vi "LVClass_ClosedLoopSecurity_Dtor.vi"(0 "ClosedLoopSecurity in":refnum<class "ClosedLoopSecurity.lvclass">, 11 "error in (no error)":errorcluster) -> (4 "ClosedLoopSecurity out":refnum<class "ClosedLoopSecurity.lvclass">, 15 "error out":errorcluster)   [LabVIEW 2020, in "ClosedLoopSecurity.lvclass"]
doc: "Destruction.\n\n<B>security_paramsIn</B> : Pointer to threaded loop object.\n<B>security_paramsOut</B> : Pointer to threaded loop object."
uses:
  ClosedLoopSecurity.lvclass
  ClosedLoopSecurity.lvclass/ClosedLoopSecurity.ctl
  Controls/Handle creation.ctl
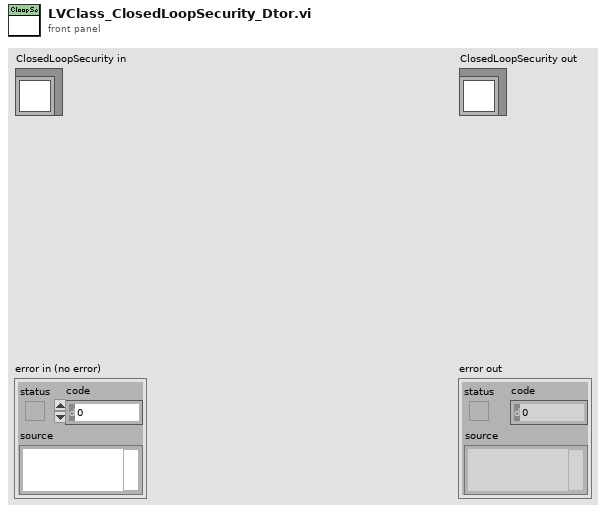
[diagram p1: front panel]
types:
  T1 = typedef "Handle creation.ctl" = enum16{"By ctor", "By write function"}
  T2 = typedef "ClassID.ctl" = i64
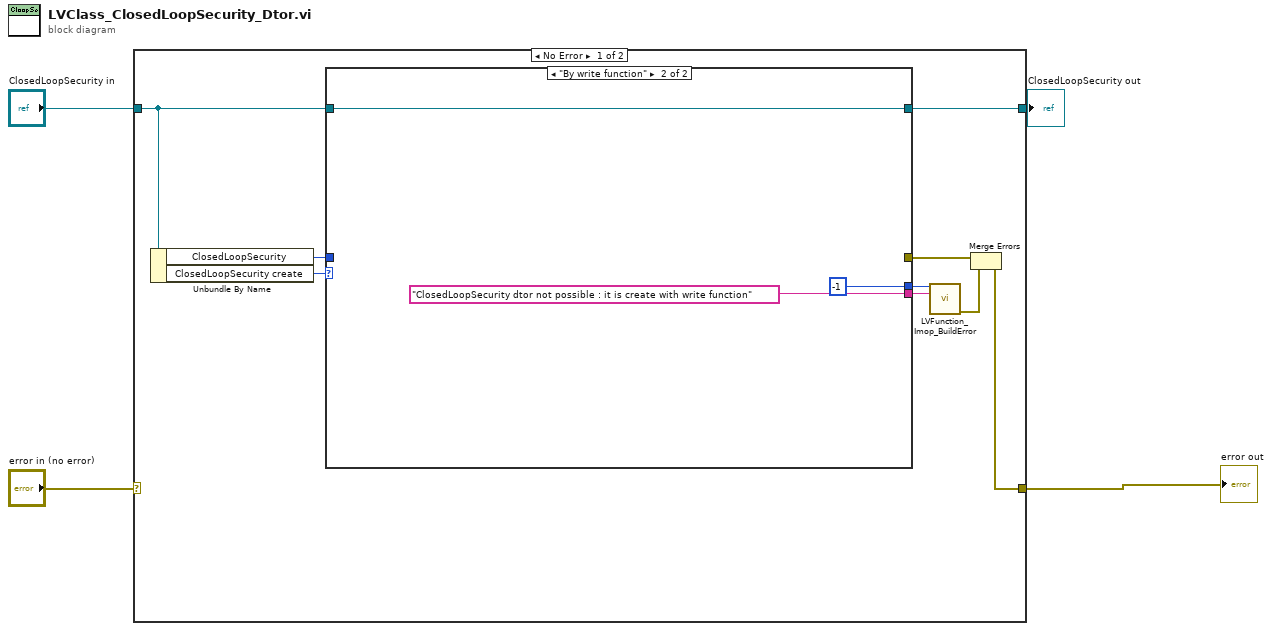
[diagram p0: block diagram]
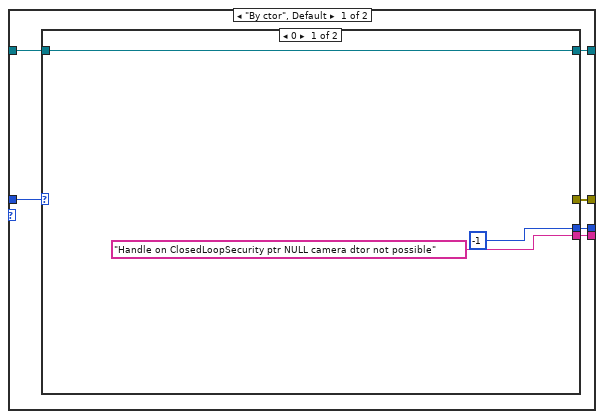
[diagram p2: hidden frame]
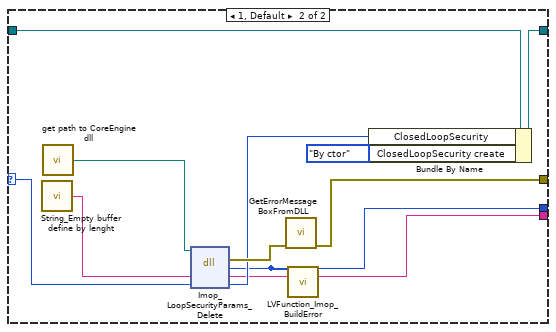
[diagram p3: hidden frame]
diagram:
  n1 = case shown="No Error" "error in (no error)" {
    selector: "error in (no error)" -> [_ w38]
    tunnel: [w5 w38] -> w3
    tunnel: [w13 w37] -> w1
    tunnel: "ClosedLoopSecurity in" -> [w12 w37]
    frame No Error {
      n2 = Unbundle By Name(w12) -> ("ClosedLoopSecurity"=w11:T2, "ClosedLoopSecurity create"=w10:T1)
      n3 = case shown="\"By write function\"" w10 {
        tunnel: [w19 w36] -> w13
        tunnel: w12 -> [w18 w36]
        tunnel: w11 -> [w17 _]
        tunnel: [w15 -1] -> w9
        tunnel: [w14 "ClosedLoopSecurity dtor not possible : it is create with write function" ("message")] -> w8
        tunnel: [w16 _] -> w6
        frame "By ctor", Default {
          n4 = case shown="0" w17 {
            selector: w17 -> [_ w23]
            tunnel: [w22 w28] -> w19
            tunnel: w18 -> [w22 w27]
            tunnel: [_ w26] -> w16
            tunnel: [-1 w25] -> w15
            tunnel: ["Handle on ClosedLoopSecurity ptr NULL camera dtor not possible" ("message") w24] -> w14
            frame 0 {
            }
            frame 1, Default {
              n5 = call "String_Empty buffer define by lenght.vi"() -> ("Empty buffer"=w33:string)  [unwired: 1 in]
              n6 = call "get path to CoreEngine dll.vi"() -> ("path to wavekit library"=w29:path)  [unwired: 14 in, 1 out]
              n7 = dll-call lib="D:/soft/HASO_v3/SVN_trunk/ImOpCoreEngine4_LV2011/DLLs/c_interface_vc100.dll" fn="Imop_LoopSecurityParams_Delete"(path in=w29, "message"=w33, "security_params"=w23) -> (error out=w32:errorcluster, "return type"=w25:i32, "message"=w24:string, "security_params"=w31:i64)  [unwired: 2 in, 1 out]
              n8 = call "GetErrorMessageBoxFromDLL.vi"("error IN"=w32) -> ("error OUT"=w26:errorcluster)  [unwired: 10 in]
              n9 = call "LVFunction_Imop_BuildError.vi"("code"=w25, "String to Prepend to source (\"\")"=w24) -> ()  [unwired: 13 in, 1 out]
              n10 = Bundle By Name(cluster=w27, "ClosedLoopSecurity"=w31, "ClosedLoopSecurity create"=Handle_creation."By ctor" ("Pupil ptr create")) -> (w28:refnum<class "ClosedLoopSecurity.lvclass">)
            }
          }
        }
        frame "By write function" {
        }
      }
      n11 = call "LVFunction_Imop_BuildError.vi"("code"=w9, "String to Prepend to source (\"\")"=w8) -> ("error out"=w7:errorcluster)  [unwired: 13 in]
      n12 = Merge Errors(w6, w7) -> (w5:errorcluster)
    }
    frame Error {
    }
  }
  "error out" <- w3
  "ClosedLoopSecurity out" <- w1
